vi "AWS-S3-BeginUpload.vi"(0 "AWS-S3-API":refnum<class "AWS-S3-API.lvclass">, 2 "Timeout (3600000msec=1hr)":i32=3600000 format="%dmsec", 5 "Object Key":string, 7 "Object Bucket":string, 9 "Source Filepath (Local)":path, 11 "error in":errorcluster, 12 "Metadata":T1[](array[typedef]), 13 "ReadWriteTimeout (3600000msec=1hr)":i32=3600000 format="%dmsec") -> (4 "AWS-S3-API out":refnum<class "AWS-S3-API.lvclass">, 8 "Object Download URL":string, 10 "Object Size (MB)":string, 15 "error out":errorcluster)   [LabVIEW 2012, in "AWS-S3-API.lvclass"]
uses:
  AWS-S3-API.lvclass
  C:/Users/Jack/repo/aws/AWS-SDK/AWSSDK.dll
  repo/aws/AWS-SDK/AWSSDK.dll
  AWS-S3-Transfer-Progress.ctl
  AWS-S3-Transfer-Header.ctl
  AWS Shared/AWS-Shared-MetadataKeyValuePair.ctl
panel:
  # "Inputs"
  # "Outputs"
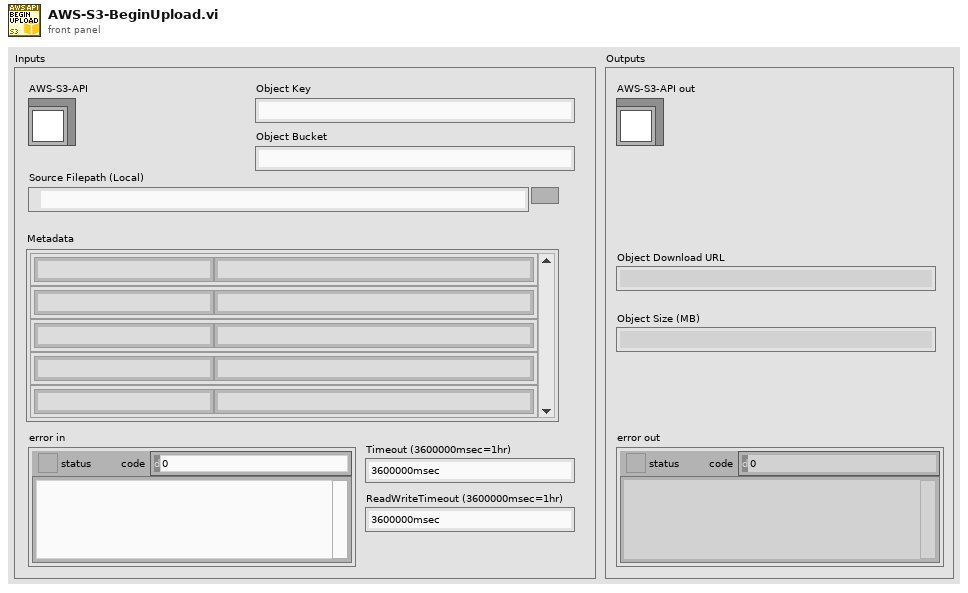
[diagram p1: front panel]
types:
  T1 = typedef "AWS-Shared-MetadataKeyValuePair.ctl" = cluster{"Key":string, "Value":string}
  T2 = cluster{"Initial Timestamp":u32, "Transfer Progress":refnum<user-event>}
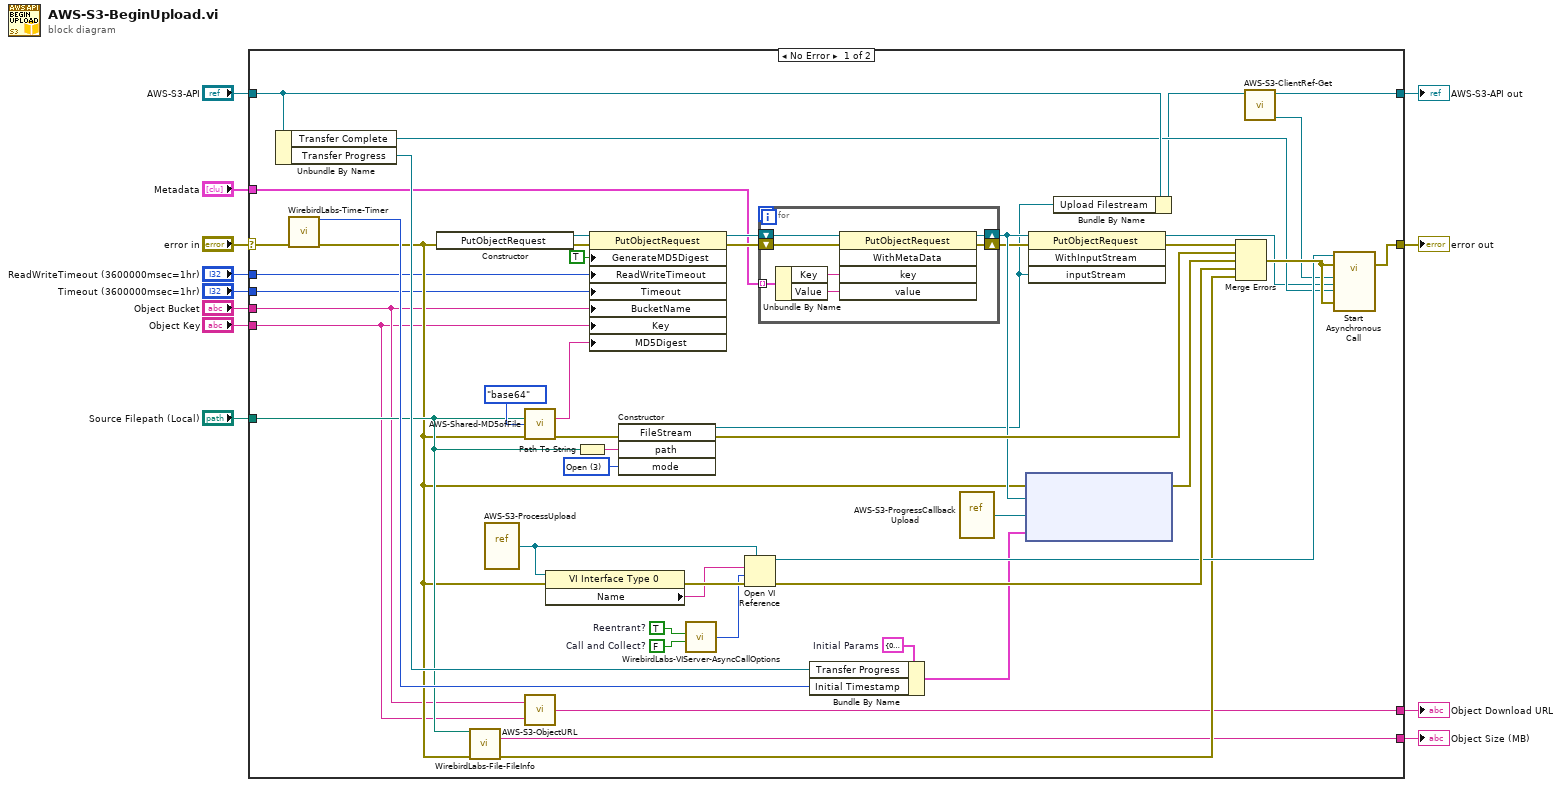
[diagram p0: block diagram]
diagram:
  n1 = case shown="No Error" "error in" {
    selector: "error in" -> [w29 w69]
    tunnel: [w26 w69] -> w12
    tunnel: [w19 w68] -> w10
    tunnel: "AWS-S3-API" -> [w54 w68]
    tunnel: "Source Filepath (Local)" -> [w25 _]
    tunnel: "Object Key" -> [w14 _]
    tunnel: "Object Bucket" -> [w15 _]
    tunnel: "Metadata" -> [w46 _]
    tunnel: [w13 _] -> w4
    tunnel: [w22 _] -> w3
    tunnel: "ReadWriteTimeout (3600000msec=1hr)" -> [w17 _]
    tunnel: "Timeout (3600000msec=1hr)" -> [w16 _]
    frame No Error {
      w31 = FALSE  # Call and Collect?
      w32 = TRUE  # Reentrant?
      w34 = 3 items=["CreateNew"=1, "Create"=2, "Open"=3, "OpenOrCreate"=4, "Truncate"=5, "Append"=6] ("mode")
      w45 = T2 {"Initial Timestamp"=0, "Transfer Progress"=refnum}  # Initial Params
      n2 = Unbundle By Name(w54) -> ("Transfer Complete"=w40:refnum<user-event>, "Transfer Progress"=w57:refnum<user-event>)
      n3 = call "WirebirdLabs-Time-Timer.vi"("error in"=w29) -> ("Timer (msec)"=w28:u32, "error out"=w24:errorcluster)  [unwired: 10 in, 3 out]
      n4 = constructor class="PutObjectRequest"(error in=w24) -> (reference out=w49:refnum<k24>, error out=w55:errorcluster)  [unwired: 2 in, 1 out]
      n5 = call "WirebirdLabs-File-FileInfo.vi"("Filepath"=w25, "error in"=w24) -> ("Filesize (MB)"=w22:string, "error out"=w23:errorcluster)  [unwired: 12 in]
      n6 = vi-ref "AWS-S3-ProcessUpload.vi"() -> (w50:refnum<vi>)
      n7 = call "AWS-Shared-MD5ofFile.vi"("Local Filepath"=w25, "Encoding"=enum16{"base64", "ASCII Hex"}."base64", "error in"=w24) -> ("MD5"=w43:string, "error out"=w33:errorcluster)  [unwired: 11 in]
      n8 = call "AWS-S3-ObjectURL.vi"("Object Bucket"=w15, "Object Key"=w14) -> ("Object URL"=w13:string)  [unwired: 2 in]
      n9 = property class="VI Interface Type 0"(reference=w50, error in=w24) -> (error out=w52:errorcluster, "Name"=w51:string)  [unwired: 1 out]
      n10 = Path To String(path=w25) -> (string=w35:string)
      n11 = property class="PutObjectRequest"(reference=w49, error in=w55, "GenerateMD5Digest"=TRUE, "ReadWriteTimeout"=w17, "Timeout"=w16, "BucketName"=w15, "Key"=w14, "MD5Digest"=w43) -> (reference out=w48:refnum<k24>, error out=w47:errorcluster)
      n12 = constructor class="FileStream"(error in=w33, "path"=w35, "mode"=w34) -> (reference out=w27:refnum<k24>, error out=w58:errorcluster)  [unwired: 2 in, 3 out]
      n13 = call "WirebirdLabs-VIServer-AsyncCallOptions.vi"("Call and Collect?"=w31, "Reentrant?"=w32) -> ("Open VI Ref Options"=w30:i32)  [unwired: 4 in]
      n14 = Open VI Reference(type specifier VI Refnum (for type only)=w50, vi path=w51, options=w30, error in (no error)=w52) -> (vi reference=w53:refnum<vi>, error out=w60:errorcluster)  [unwired: 2 in]
      n15 = for {
        shift-right: [w64] -> w39
        shift-left: w48 -> [w67]
        shift-right: [w65] -> w38
        shift-left: w47 -> [w66]
        tunnel: w46 -> [w63] mode=indexing
        n16 = Unbundle By Name(w63) -> ("Key"=w62:string, "Value"=w61:string)
        n17 = invoke class="PutObjectRequest" method="WithMetaData"(reference=w67, error in=w66, "key"=w62, "value"=w61) -> (reference out=w64:refnum<k24>, error out=w65:errorcluster)  [unwired: 1 in, 3 out]
      }
      n18 = Bundle By Name(cluster=w45, "Transfer Progress"=w57, "Initial Timestamp"=w28) -> (w44:T2)
      n19 = vi-ref "AWS-S3-ProgressCallbackUpload.vi"() -> ("vi reference"=w41:refnum<vi>)
      n20 = node(w24, w39, w41, w44) -> (w59:errorcluster)  [unwired: 1 in, 1 out]
      n21 = invoke class="PutObjectRequest" method="WithInputStream"(reference=w39, error in=w38, "inputStream"=w27) -> (reference out=w36:refnum<k24>, error out=w37:errorcluster)  [unwired: 1 in, 2 out]
      n22 = Bundle By Name(cluster=w54, "Upload Filestream"=w27) -> (w20:refnum<class "AWS-S3-API.lvclass">)
      n23 = Merge Errors(w37, w58, w59, w60, w23) -> (w56:errorcluster)
      n24 = call "AWS-S3-ClientRef-Get.vi"("AWS-S3-API"=w20) -> ("S3 Client ref"=w21:refnum<k24>, "AWS-S3-API out"=w19:refnum<class "AWS-S3-API.lvclass">)  [unwired: 9 in]
      n25 = call-by-ref "Start Asynchronous Call"(reference=w53, error in=w56, "S3 Client ref"=w21, "Put Object Request ref"=w36, "Upload Complete"=w40, "error in"=w56) -> (error out=w26:errorcluster)  [unwired: 12 in, 1 out]
    }
    frame Error {
    }
  }
  "error out" <- w12
  "AWS-S3-API out" <- w10
  "Object Download URL" <- w4
  "Object Size (MB)" <- w3
